vi "System Health and Monitoring.vi"(11 "queue in":refnum<queue>) -> ()   [LabVIEW 2014]
uses:
  C:/Users/Sam/OneDrive/Github/MyRIO-Robot/controls/UI Data.ctl
  <vilib>/nisyscfg/Close (System).vi
  <vilib>/nisyscfg/nisyscfg.lvlib
  <vilib>/NI_Real-Time Target Support.lvlib
  <resource>/objmgr/nisysapi.rc
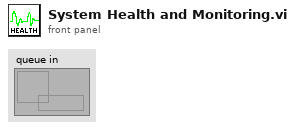
[diagram p1: front panel]
types:
  T1 = typedef "NI_Real-Time Target Support.lvlib/RT CPU Load.ctl" = cluster{"Total (%)":dbl, "Time Critical (%)":dbl, "Timed Structures (%)":dbl, "High (%)":dbl, "Above Normal (%)":dbl, "Normal (%)":dbl, "Background (%)":dbl, "Idle (%)":dbl, "ISR (%)":dbl}
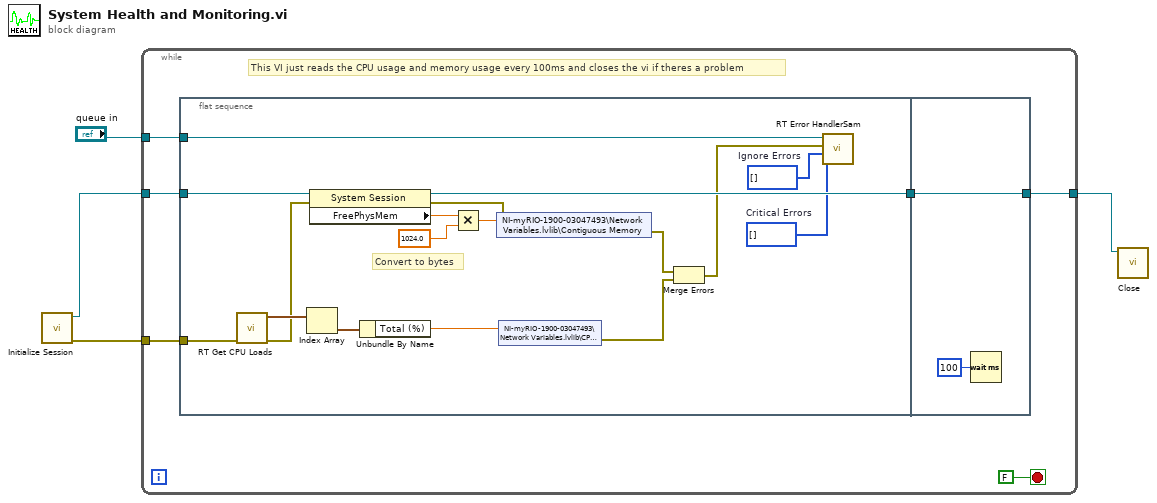
[diagram p0: block diagram]
diagram:
  n1 = call <vilib>:"Initialize Session.vi"() -> ("error out"=w4:errorcluster, "Session out"=w3:refnum<k21>)  [unwired: 10 in]
  n2 = while {
    tunnel: w4 -> [w10]
    tunnel: w3 -> [w9]
    tunnel: [w6] -> w2
    tunnel: "queue in" -> [w5]
    stop <- FALSE stop-if-true
    # "This VI just reads the CPU usage and memory usage every 100ms and closes the vi if theres a problem"
    n3 = flat-sequence {
      tunnel: w10 -> [w27]
      tunnel: w9 -> [w24]
      tunnel: [w15] -> w8
      tunnel: w5 -> [w14]
      tunnel: w8 -> [w28]
      tunnel: [w28] -> w6
      frame #0 {
        w11 = i32[] []  # Ignore Errors
        w12 = i32[] []  # Critical Errors
        # "Convert to bytes"
        n4 = call <vilib>:"RT Get CPU Loads.vi"("error in (no error)"=w27) -> ("error out"=w23:errorcluster, "CPU loads"=w26:T1[])  [unwired: 9 in]
        n5 = Index Array(array=w26) -> (element=w25:T1)  [unwired: 1 in]
        n6 = property class="System Session"(reference=w24, error in=w23) -> (reference out=w15:refnum<k21>, error out=w19:errorcluster, "FreePhysMem"=w22:dbl)
        n7 = Unbundle By Name(w25) -> ("Total (%)"=w18:dbl)
        n8 = Multiply(x=w22, y=1024.0) -> (x*y=w20:dbl)
        n9 = shared-variable "NI-myRIO-1900-03047493\\Network Variables.lvlib\\Contiguous Memory"(w20, error in=w19) -> (error out=w17:errorcluster)
        n10 = shared-variable "NI-myRIO-1900-03047493\\Network Variables.lvlib\\CPU Usage"(w18) -> (error out=w16:errorcluster)  [unwired: 1 in]
        n11 = Merge Errors(w17, w16) -> (w13:errorcluster)
        n12 = call "RT Error HandlerSam.vi"("Ignore Errors"=w11, "Critical Errors"=w12, "error to process"=w13, "queue in"=w14) -> ()  [unwired: 7 in, 1 out]
      }
      frame #1 {
        n13 = Wait (ms)(milliseconds to wait=u32 100) -> ()  [unwired: 1 out]
      }
    }
  }
  n14 = call-poly <vilib>:"Close.vi"("Session in"=w2) -> ()  [unwired: 10 in, 1 out]
